vi "PDSS - New Trigger Sequence - FLCs and Trigger are Delayed from LCVRs.vi"(7 "Modulation Cycles per Wavelength":dbl=1.0 min=1.0 max=30.0 step=1.0, 8 "error in":errorcluster, 10 "FPS":dbl=30.0 min=0.01 max=49.0 step=1.0 format="%0.2p", 11 "LCVR Tuning Voltages":dbl[](array[numeric])=[1.0, 1.1, 1.2000000000000002, 1.3000000000000003] format="%.3g") -> (0 "error out":errorcluster, 1 "LCVR Relaxtion Time (ms)":dbl=200.0 format="%#_13g", 2 "AO Waveforms":waveform(dbl)[](array[waveform])=[{"t0"=timestamp(0 s since 1904-01-01), "dt"=0.000125, "Y"=array[3200 elements]}, {"t0"=timestamp(0 s since 1904-01-01), "dt"=0.000125, "Y"=array[3200 elements]}, {"t0"=timestamp(0 s since 1904-01-01), "dt"=0.000125, "Y"=array[3200 elements]}, {"t0"=timestamp(0 s since 1904-01-01), "dt"=0.000125, "Y"=array[3200 elements]}, {"t0"=timestamp(0 s since 1904-01-01), "dt"=0.000125, "Y"=array[3200 elements]}, {"t0"=timestamp(0 s since 1904-01-01), "dt"=0.000125, "Y"=array[3200 elements]}, {"t0"=timestamp(0 s since 1904-01-01), "dt"=0.000125, "Y"=array[3200 elements]}, {"t0"=timestamp(0 s since 1904-01-01), "dt"=0.000125, "Y"=array[3200 elements]}], 3 "True Camera Exposure":dbl)   [LabVIEW 2014]
doc: "Nematic LC's require a modulation frequency of 2 kHz. If we sample each period with 4 samples, this means a sampling rate of 8000 samples per second = 125 microseconds per update\n\nThe default acquisition sequence is a \"Wavelength Tuning Relaxation Delay\" wherein no images are being acquired followed by a \"Wavelength Acquisition Interval\".\nThis is then repeated for 'n' wavelength intervals (typically 3 or 5)."
uses:
  <vilib>/Waveform/WDTOps.llb/WDT Append Waveforms DBL.vi
  <vilib>/measure/NI_MABase.lvlib
panel:
  out "Trigger Duty Cycle":dbl
  out "AO Graph":waveform(dbl)[](graph)=[{"t0"=timestamp(0 s since 1904-01-01), "dt"=0.000125, "Y"=array[3200 elements]}, {"t0"=timestamp(0 s since 1904-01-01), "dt"=0.000125, "Y"=array[3200 elements]}, {"t0"=timestamp(0 s since 1904-01-01), "dt"=0.000125, "Y"=array[3200 elements]}, {"t0"=timestamp(0 s since 1904-01-01), "dt"=0.000125, "Y"=array[3200 elements]}, {"t0"=timestamp(0 s since 1904-01-01), "dt"=0.000125, "Y"=array[3200 elements]}, {"t0"=timestamp(0 s since 1904-01-01), "dt"=0.000125, "Y"=array[3200 elements]}, {"t0"=timestamp(0 s since 1904-01-01), "dt"=0.000125, "Y"=array[3200 elements]}, {"t0"=timestamp(0 s since 1904-01-01), "dt"=0.000125, "Y"=array[3200 elements]}]
  # "User Adjustable Values are in this box"
  # "We've decided (Matus and Scott) to just use external triggered mode acquisition.  \nIn this mode, the rising edge of the trigger pulse initiates the\ncamera exposure but the duration of the exposure is controlled by a pre-set camera clock.  \nTherefore duty cycle for the trigger waveform generation is not important.\n\n13-Nov-2013 - The delay before each wavelength interval is 2 sets of modulation cyles (2 x 133 ms = 266 ms)\n\nThis is because we're starting the modulation waveforms at the same time as we start the trigger delay and\nthe required time for 1 modulation cycle is 4 x 33.33 ms = 133 ms.  In one modulation cycle, the LCVR's still\nwon't have completely tuned to the correct desired wavelength.\n\nIf we want to regain these 66 ms, we can delay the start of the modulation pulses to begin exactly at 200ms\n\n\nThis sequence depends on the exposure time being set to 33.3ms\n\nThe Goodrich Camera OPR Setting 22 produces an exposure (internally timed) of 31.994 ms.\nEach modulation state lasts 33.3 ms therefore the duty cycle of the trigger square is 31.994/33.3333 = 96%\n\nIt is important to have the phase be low enought so that there is not an articifial trigger pulse (this occurs at a phase of -15)\n\nWe've determined that a phase of -10 degrees and a duty cycle of 96% produce a camera exposure that lies entirely\nwithin a single modulation state."
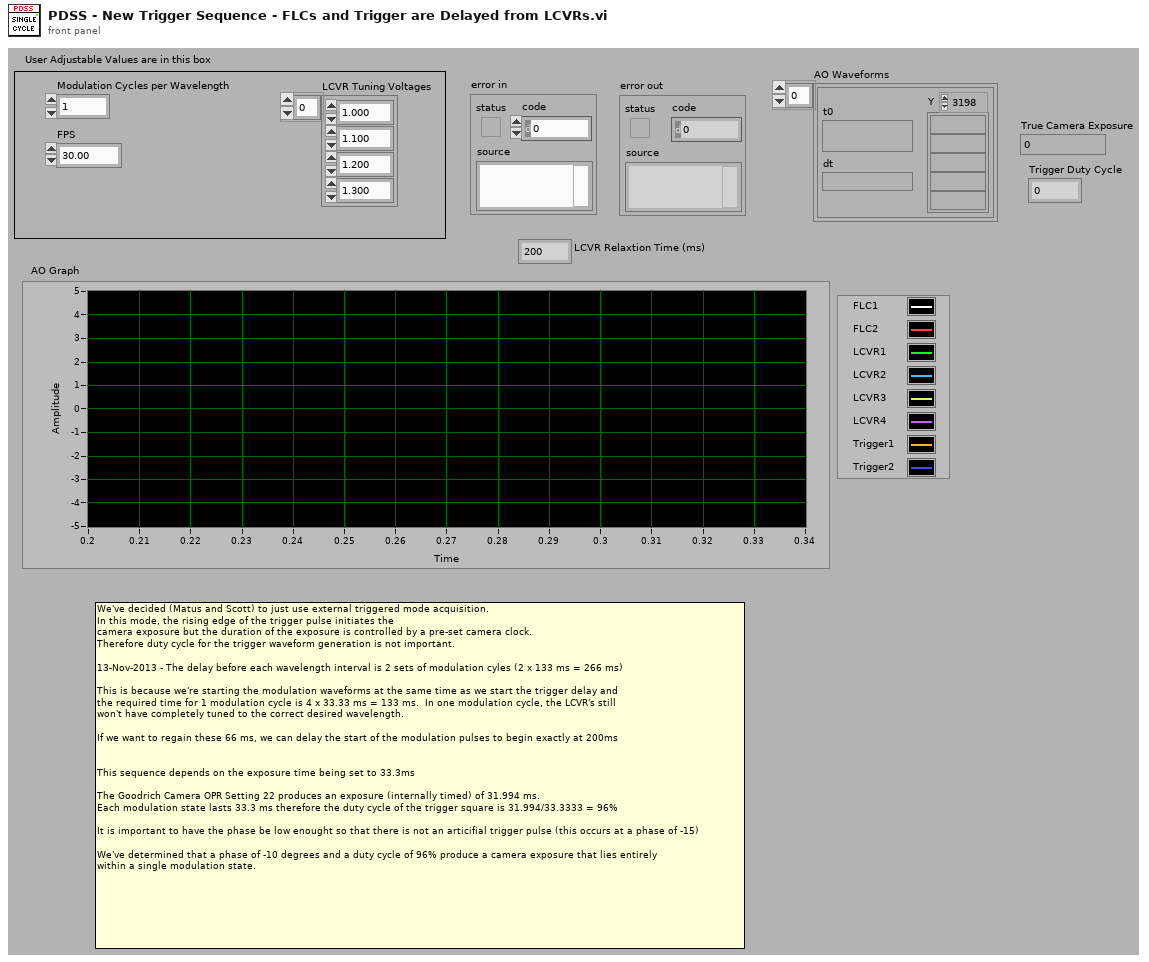
[diagram p1: front panel]
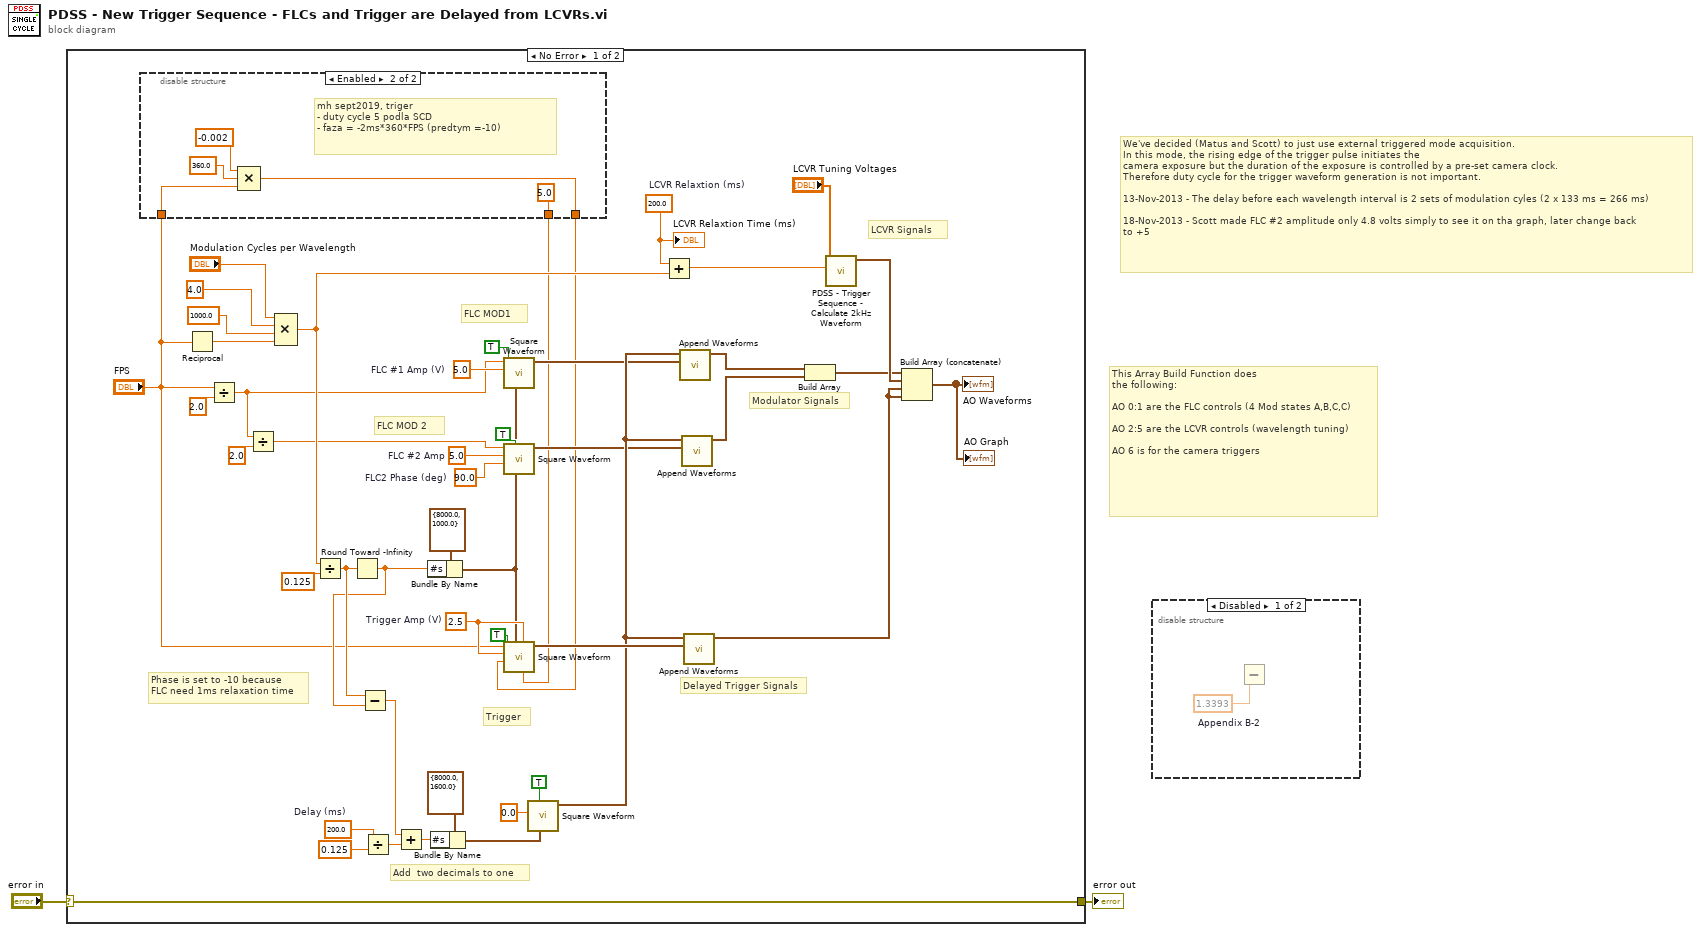
[diagram p0: block diagram]
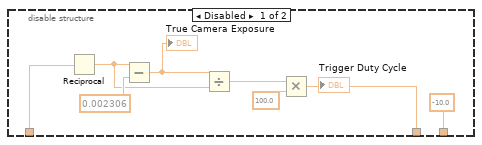
[diagram p3: hidden frame]
diagram:
  # "We've decided (Matus and Scott) to just use external triggered mode acquisition.  \nIn this mode, the rising edge of the trigger pulse initiates the\ncamera exposure but the duration of the exposure is controlled by a pre-set camera clock.  \nTherefore duty cycle for the trigger waveform generation is not important.\n\n13-Nov-2013 - The delay before each wavelength interval is 2 sets of modulation cyles (2 x 133 ms = 266 ms)\n\n18-Nov-2013 - Scott made FLC #2 amplitude only 4.8 volts simply to see it on tha graph, later change back\nto +5"
  # "This Array Build Function does\nthe following:\n\nAO 0:1 are the FLC controls (4 Mod states A,B,C,C)\n\nAO 2:5 are the LCVR controls (wavelength tuning)\n\nAO 6 is for the camera triggers"
  n1 = case shown="No Error" "error in" {
    selector: "error in" -> [w49 w63]
    tunnel: [w49 w63] -> w1
    frame No Error {
      w13 = 200.0  # LCVR Relaxtion (ms)
      w28 = 200.0  # Delay (ms)
      w32 = 2.5  # Trigger Amp (V)
      w38 = 5.0  # FLC #2 Amp
      w45 = 5.0  # FLC #1 Amp (V)
      w48 = 90.0  # FLC2 Phase (deg)
      # "FLC MOD 2"
      # "FLC MOD1"
      # "Trigger"
      # "Phase is set to -10 because \nFLC need 1ms relaxation time"
      # "Add  two decimals to one"
      # "Delayed Trigger Signals"
      # "LCVR Signals"
      # "Modulator Signals"
      n2 = disable-structure shown="Enabled" {
        disable-tunnel: "FPS" -> [w57 w59]
        disable-tunnel: [w51 5.0 ("duty cycle (%)")] -> w7
        disable-tunnel: [-10.0 ("phase") w58] -> w6
        frame Disabled {
          n3 = Reciprocal(x=w57) -> (1/x=w54:dbl)
          n4 = Subtract(x=w54, y=0.002306) -> (x-y=w55:dbl)
          "True Camera Exposure" <- w55
          n5 = Divide(x=w55, y=w54) -> (x/y=w53:dbl)
          n6 = Multiply(x=w53, y=100.0) -> (x*y=w51:dbl)
          "Trigger Duty Cycle" <- w51
        }
        frame Enabled {
          # "mh sept2019, triger \n- duty cycle 5 podla SCD\n- faza = -2ms*360*FPS (predtym =-10)"
          n7 = Compound Arithmetic op=MULTIPLY(-0.002 ("value"), 360.0 ("value"), w59) -> (w58:dbl)
        }
      }
      n8 = Reciprocal(x="FPS") -> (1/x=w12:dbl)
      n9 = Divide(x="FPS", y=2.0) -> (x/y=w4:dbl)
      n10 = Divide(x=w4, y=2.0) -> (x/y=w3:dbl)
      n11 = Compound Arithmetic op=MULTIPLY("Modulation Cycles per Wavelength", 4.0 ("Mod States Per Interval"), 1000.0 ("x"), w12) -> (w8:dbl)
      n12 = Divide(x=w8, y=0.125) -> (x/y=w40:dbl)
      n13 = Round Toward -Infinity(1:w40) -> (0:w39:dbl)
      n14 = Subtract(x=w40, y=w39) -> (x-y=w24:dbl)
      n15 = Divide(x=w28, y=0.125) -> (x/y=w26:dbl)
      n16 = Add(x=w24, y=w26) -> (x+y=w25:dbl)
      n17 = Bundle By Name(cluster=cluster{"Fs":dbl, "#s":dbl} {"Fs"=8000.0, "#s"=1000.0} ("sampling info"), "#s"=w39) -> (w16:cluster{"Fs":dbl, "#s":dbl})
      n18 = Bundle By Name(cluster=cluster{"Fs":dbl, "#s":dbl} {"Fs"=8000.0, "#s"=1600.0} ("sampling info"), "#s"=w25) -> (w30:cluster{"Fs":dbl, "#s":dbl})
      n19 = call <vilib>:"Square Waveform.vi"("sampling info"=w16, "reset signal"=TRUE, "amplitude"=w45, "frequency"=w4) -> ("signal out"=w20:waveform(dbl))  [unwired: 6 in, 1 out]
      n20 = call <vilib>:"Square Waveform.vi"("sampling info"=w16, "reset signal"=TRUE, "phase"=w48, "amplitude"=w38, "frequency"=w3) -> ("signal out"=w18:waveform(dbl))  [unwired: 5 in, 1 out]
      n21 = call <vilib>:"Square Waveform.vi"("duty cycle (%)"=w7, "offset"=w32, "sampling info"=w16, "reset signal"=TRUE, "phase"=w6, "amplitude"=w32, "frequency"="FPS") -> ("signal out"=w27:waveform(dbl))  [unwired: 3 in, 1 out]
      n22 = call <vilib>:"Square Waveform.vi"("sampling info"=w30, "reset signal"=TRUE, "amplitude"=0.0 ("Delay Voltage (no triggers)")) -> ("signal out"=w21:waveform(dbl))  [unwired: 7 in, 1 out]
      n23 = Add(x=w13, y=w8) -> (x+y=w15:dbl)
      n24 = call-poly <vilib>:"Append Waveforms.vi"("waveform B"=w20, "waveform A"=w21) -> ("waveform out"=w19:waveform(dbl))  [unwired: 8 in, 1 out]
      n25 = call-poly <vilib>:"Append Waveforms.vi"("waveform B"=w18, "waveform A"=w21) -> ("waveform out"=w17:waveform(dbl))  [unwired: 8 in, 1 out]
      n26 = call-poly <vilib>:"Append Waveforms.vi"("waveform B"=w27, "waveform A"=w21) -> ("waveform out"=w41:waveform(dbl))  [unwired: 8 in, 1 out]
      n27 = Build Array(w19, w17) -> (w44:waveform(dbl)[])
      n28 = call "PDSS - Trigger Sequence - Calculate 2kHz Waveform.vi"("Time (200 ms)"=w15, "Voltages"="LCVR Tuning Voltages") -> ("tuning waveforms"=w47:waveform(dbl)[])  [unwired: 8 in, 1 out]
      n29 = Build Array (concatenate)(w44, w47, w41, w41) -> (→"AO Waveforms" →"AO Graph":waveform(dbl)[])
      "LCVR Relaxtion Time (ms)" <- w13
    }
    frame Error {
    }
  }
  "error out" <- w1
  n30 = disable-structure shown="Disabled" {
    frame Disabled {
      w64 = 1.3393  # Appendix B-2
      n31 = Subtract(y=w64) -> ()  [unwired: 1 in, 1 out]
    }
    frame Enabled {
    }
  }
